vi "创建虎对象.vi"() -> (3 "Animal输出":refnum<class "tiger.lvclass">)   [LabVIEW 2020, in "tiger.lvclass"]
uses:
  tiger.lvclass
  Animal/Animal.lvclass/Animal.ctl
  Animal/Animal.lvclass
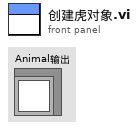
[diagram p1: front panel]
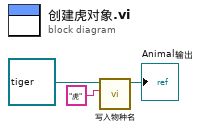
[diagram p0: block diagram]
diagram:
  n1 = call "写入物种名.vi"("物种名"="虎", "Animal输入"=refnum<class "tiger.lvclass"> refnum ("tiger.lvclass")) -> ("Animal输出"=→"Animal输出":refnum<class "tiger.lvclass">)  [unwired: 8 in, 1 out]
